vi "Write Associated Controller Actor Name.vi"(8 "error in (no error)":errorcluster, 10 "Associated Controller Actor Name":string, 11 "CS++GUIActor in":refnum<class "CS++GUIActor.lvclass">) -> (0 "error out":errorcluster, 3 "CS++GUIActor out":refnum<class "CS++GUIActor.lvclass">)   [LabVIEW 2014, in "CS++GUIActor.lvlib" / "CS++GUIActor.lvclass"]
uses:
  CS++GUIActor.lvclass
  CS++GUIActor.lvclass/CS++GUIActor.ctl
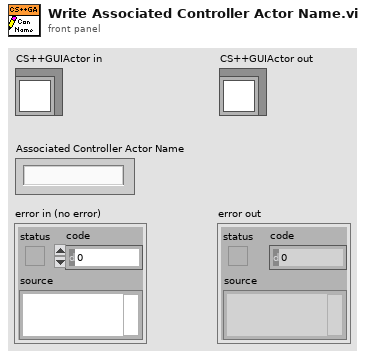
[diagram p1: front panel]
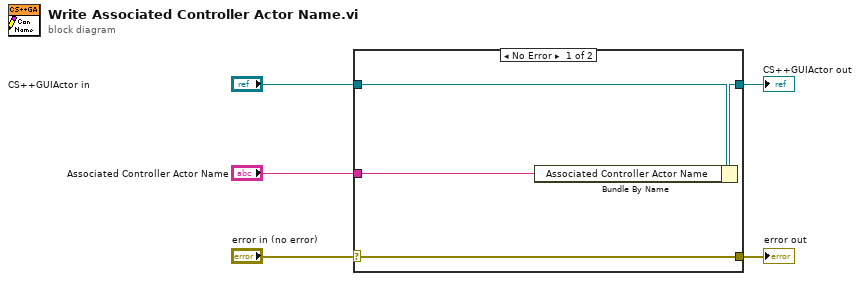
[diagram p0: block diagram]
diagram:
  n1 = case shown="No Error" "error in (no error)" {
    selector: "error in (no error)" -> [w9 w10]
    tunnel: [w9 w10] -> w4
    tunnel: [w7 w11] -> w2
    tunnel: "CS++GUIActor in" -> [w8 w11]
    tunnel: "Associated Controller Actor Name" -> [w6 _]
    frame No Error {
      n2 = Bundle By Name(cluster=w8, "Associated Controller Actor Name"=w6) -> (w7:refnum<class "CS++GUIActor.lvclass">)
    }
    frame Error {
    }
  }
  "error out" <- w4
  "CS++GUIActor out" <- w2
